vi "Append Execution Units List.vi"(0 "Input List":string[](array[string]), 1 "Item Ref":T1 format="%.0x", 5 "Input Refs":T1[](array[typedef]) format="%.0x", 7 "Execution Unit Name":string, 9 "Found?":bool) -> (4 "List Out":string[](array[string]), 6 "Ref Out":T1[](array[typedef]) format="%.0x")   [LabVIEW 2020, in "AIM ARINC 664 Scripting.lvlib"]
uses:
  AIM ARINC 664 Scripting.lvlib
  <vilib>/NI VeriStand/Custom Device API/Custom Device Item Ref.ctl
  <vilib>/NI VeriStand/Custom Device API/Custom Device API.lvlib
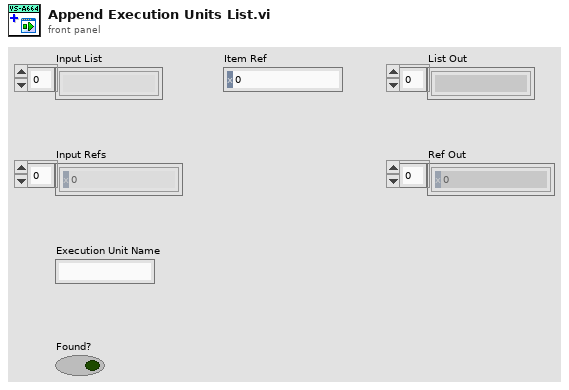
[diagram p1: front panel]
types:
  T1 = typedef "Custom Device API.lvlib/Custom Device Item Ref.ctl" = u64
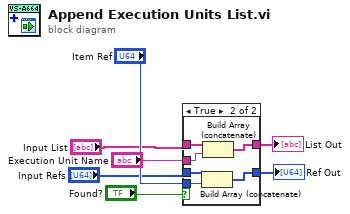
[diagram p0: block diagram]
diagram:
  n1 = case shown="True" "Found?" {
    tunnel: "Input Refs" -> [w9 w14]
    tunnel: "Input List" -> [w8 w15]
    tunnel: "Item Ref" -> [_ w13]
    tunnel: [w8 w12] -> w6
    tunnel: [w9 w11] -> w7
    tunnel: "Execution Unit Name" -> [_ w10]
    frame False {
    }
    frame True {
      n2 = Build Array (concatenate)(w14, w13) -> (w11:T1[])
      n3 = Build Array (concatenate)(w15, w10) -> (w12:string[])
    }
  }
  "Ref Out" <- w7
  "List Out" <- w6
